vi "Motor controller.vi"() -> ()   [LabVIEW 2015]
uses:
  Power control/Power control.lvclass
  <vilib>/Utility/config.llb/Write Key (Double).vi
  <vilib>/Utility/config.llb/Write Key (String).vi
  <vilib>/Utility/config.llb/Write Key (Boolean).vi
  <vilib>/Utility/config.llb/Write Key (I32).vi
  <vilib>/Utility/config.llb/Read Key (Double).vi
  <vilib>/Utility/config.llb/Read Key (String).vi
  <vilib>/Utility/config.llb/Read Key (Boolean).vi
  <vilib>/Utility/config.llb/Read Key (I32).vi
  Motor controller/Motor/Motor.lvclass
  Motor controller/Signaller/Signaller.lvclass
  Motor controller/Automatic mode/Automatic Mode.lvclass
  Motor controller/Motor/AlphaStep One/AlphaStep One.lvclass
  Motor controller/Motor/Dummy Motor/Dummy Motor.lvclass
  <vilib>/Utility/config.llb/NI_LVConfig.lvlib
  Position-Tracker/x64/Release/PositionTrackerDll.dll
  Motor-Tracker/Release/x64/MotorTrackerDll.dll
panel:
  out "error out":errorcluster
  out "Calculated\nFrequency":dbl
  in  "Show advanced configuration":bool
  in  "Tab Control":enum32{"Advanced configuration"}(tab)
  in  "Reseek after # bad":u32=4
  in  "Samples per step":i32=3 min=0
  in  "\"Good\" rate threshold":dbl=0.8 min=0.0
  out "Countdown overridden":bool
  in  "Algorithm switch time (min)":i64=10 min=0
  out "Automatic mode start":timestamp
  in  "0.01 GHz/step":bool
  in  "0.05 GHz/step":bool
  in  "0.03 GHz/step":bool
  in  "Reset everything":bool
  in  "Make up fit parameters":bool
  in  "Automatic velocity (rev/sec)":dbl=0.1 min=0.0 max=1.0
  in  "Reseek":bool
  in  "Automatic step size (rev)":dbl=0.01 min=0.0 max=1.0
  in  "Reset countdown":bool
  out "Polarization switch countdown":string="0:00"
  in  "Polarization seek":bool
  in  "Home frequency":cluster{"Positive":dbl, "Negative":dbl}={"Positive"=140.18, "Negative"=140.45} {"Negative" format="%.3g"; "Positive" format="%.3g"}
  in  "Negative seek bounds":cluster{"Minimum":dbl, "Maximum":dbl}={"Minimum"=140.35, "Maximum"=140.65} {"Maximum" format="%.3g"; "Minimum" format="%.3g"}
  in  "Positive seek bounds":cluster{"Minimum":dbl, "Maximum":dbl}={"Minimum"=140.1, "Maximum"=140.3} {"Maximum" format="%.3g"; "Minimum" format="%.3g"}
  in  "Seek positive polarization":bool=TRUE
  in  "Launch simulation":bool
  out "Polarization":dbl
  out "Eventnum":i64
  out "Samples taken":i32
  out "Rate":dbl
  in  "Data input file":path
  in  "Automatic mode on/off":bool
  in  "Add power reading":bool
  in  "Width (GHz)":dbl=0.05 format="%.3g"
  in  "New power (mW)":dbl=1.0 format="%.3g"
  out "Microwave power (mW)":dbl format="%.3g"
  in  "Home frequency 2":cluster{"Positive":dbl, "Negative":dbl}={"Positive"=140.18, "Negative"=140.45} {"Negative" format="%.3g"; "Positive" format="%.3g"}
  in  "Debug mode":bool
  in  "Stop communication":bool
  in  "COM Port":refnum<visa-resource-name>
  in  "Step size (GHz)":dbl min=0.0 max=1.0 step=0.001 format="%.3g"
  in  "Goto frequency":bool
  in  "Frequency to seek (GHz)":dbl format="%.3g"
  in  "Stop motor":bool
  in  "Move up":bool
  in  "Move down":bool
  in  "Velocity (rev/sec)":dbl min=0.0 max=1.0 step=0.001
  in  "Step size (rev)":dbl=0.01 min=0.0 max=5.0 step=0.001 format="%.3g"
  in  "Restore configuration from file":bool
  in  "Save configuration to file":bool
  in  "Refine fit parameters":bool
  out "Fit parameters":cluster{"Slope":dbl, "Intercept":dbl}
  in  "Calculate fit parameters":bool
  in  "Read position 2":bool
  in  "Read position 1":bool
  out "Position 2":dbl
  in  "Frequency 2":dbl=140.4 min=0.0 step=0.001 format="%.3g"
  out "Position 1":dbl
  in  "Frequency 1":dbl=140.0 min=0.0 step=0.001 format="%.3g"
  out "Alarm":bool
  out "Alarm code":i32 format="0x%02x"
  out "Frequency (calculated, GHz)":dbl format="%.3g"
  out "Motor position (rev)":dbl format="%.3g"
  out "Motor time (sec)":dbl
  # "Advanced configuration"
  # "Step size presets"
  # "Automatic control"
  # "Power data"
  # "Communication setup"
  # "Please wait after stopping the VI; it can take some time to shut down all the stuff running in the background, so please be patient."
  # "Manual motor control"
  # "Configuration backup/restore"
  # "The settings which are backed up by this method are: step size, frequency to seek, fit slope, fit intercept, automatic step size, automatic velocity, data input file, and all the other controls under \"Automatic control\"."
  # "Frequency calibration"
  # "Motor alarm (error)"
  # "See motor manual, section \"Troubleshooting\" for explanation of alarm codes; fix the problem first and then restart this VI"
  # "Motor information"
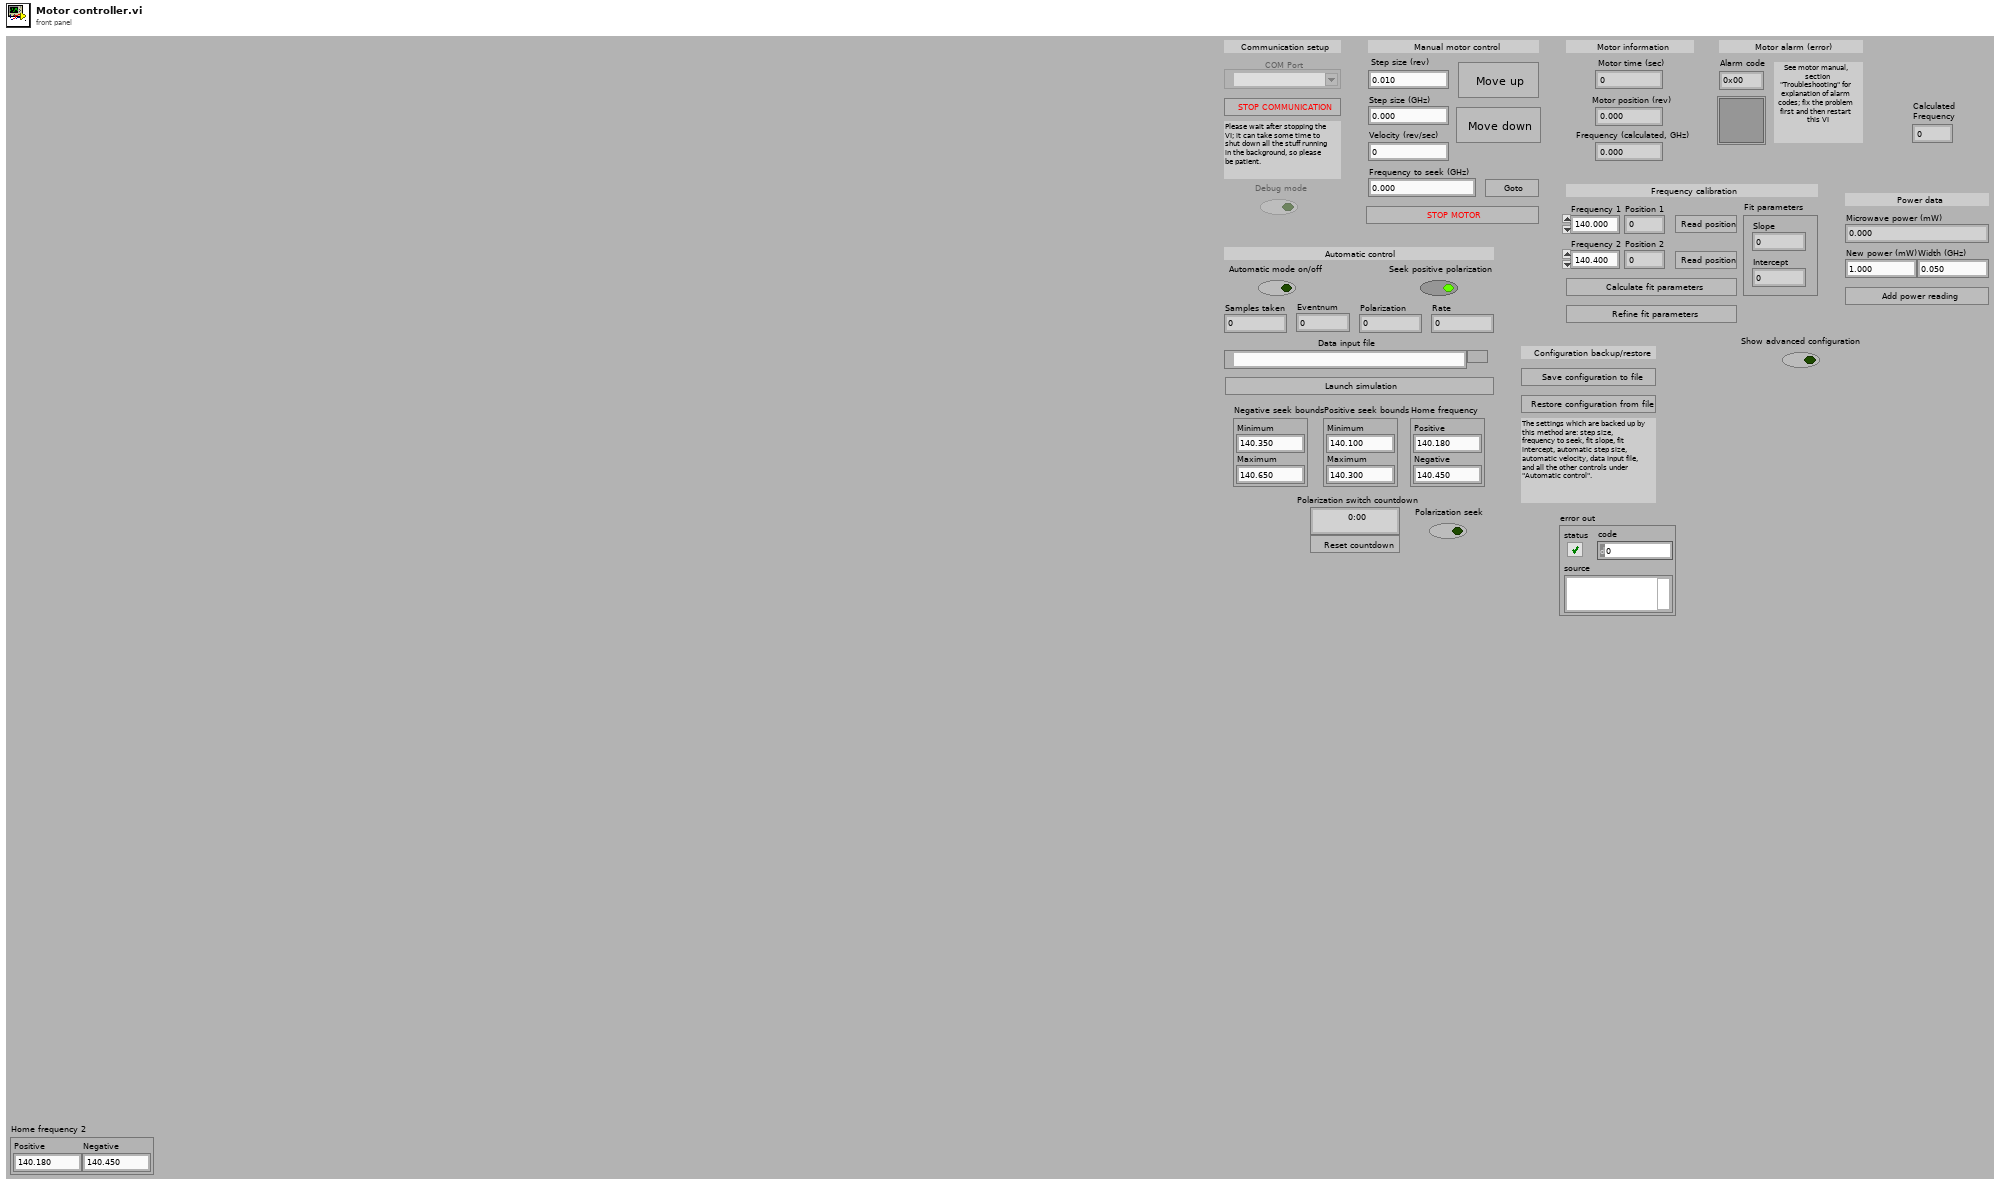
[diagram p1: front panel]
types:
  T1 = enum8{"Enabled", "Disabled", "Disabled and Grayed Out"}
  T2 = typedef "NI_LVConfig.lvlib/Config Data RefNum.ctl" = refnum<k1>
  T3 = typedef "Controller decision.ctl" = enum16{"No motion", "Switch direction", "Keep current direction"}
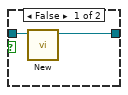
[diagram p2: hidden frame]
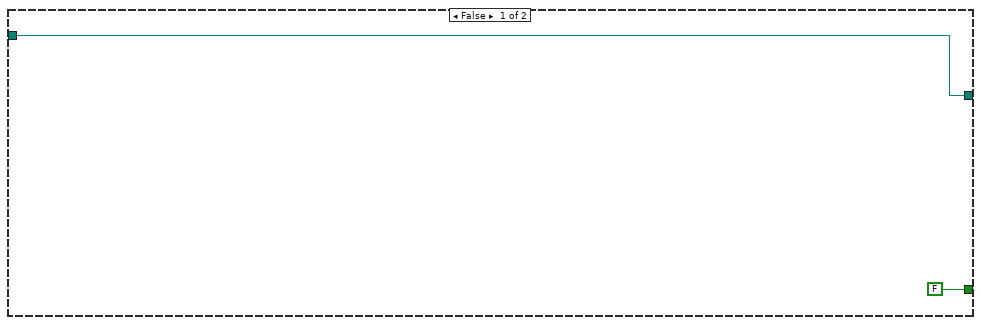
[diagram p5: hidden frame]
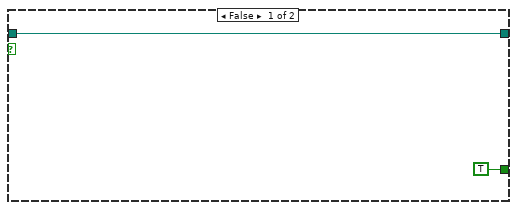
[diagram p6: hidden frame]
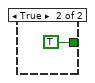
[diagram p7: hidden frame]
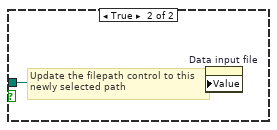
[diagram p8: hidden frame]
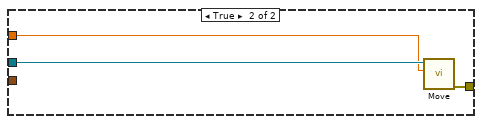
[diagram p12: hidden frame]
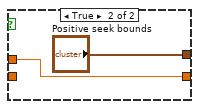
[diagram p13: hidden frame]
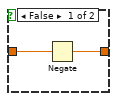
[diagram p14: hidden frame]
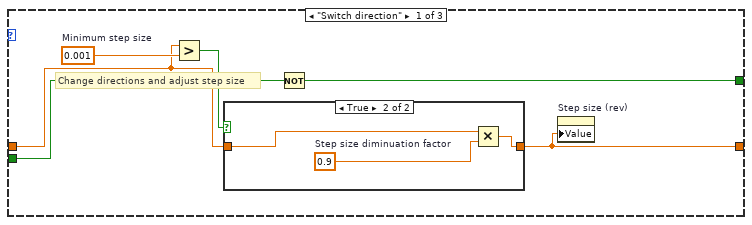
[diagram p15: hidden frame]
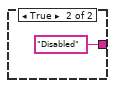
[diagram p18: hidden frame]
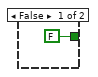
[diagram p20: hidden frame]
diagram:
  w7 = refnum<class "Power control.lvclass"> refnum  # Power control
  w41 = TRUE  # Positive direction?
  (unwired) i64 0
  # "Stop signaller"
  # "Create a new automatic mode object\nto keep track of our data"
  # "Automatic mode loop"
  n1 = Not(x="Debug mode") -> (.not. x?=w34:bool)
  n2 = Equal?(x="COM Port", y=refnum<visa-resource-name> refnum) -> (x = y?=w35:bool)
  n3 = And(x=w35, y=w34) -> (x .and. y?=w36:bool)
  n4 = case shown="True" w36 {
    tunnel: "COM Port" -> [w43 w44]
    tunnel: [w43 w44] -> w32
    frame False {
    }
    frame True {
      # "Make sure that a COM port is\nselected before trying to do\nother stuff; otherwise, bad\nthings will happen"
      n5 = call "Display Message to User5"() -> ("Got it, thanks"=w45:bool)  [unwired: 10 in, 1 out]
      n6 = Stop(stop? (T)=w45) -> ()
    }
  }
  n7 = vi-ref "Grapher.vi"() -> (w12:refnum<vi>)
  n8 = property class="VI Interface Type 3"(reference=w12) -> ("Name"=w13:string)  [unwired: 1 in, 2 out]
  n9 = Open VI Reference(type specifier VI Refnum (for type only)=w12, vi path=w13, options=128) -> (vi reference=w15:refnum<vi>)  [unwired: 3 in, 1 out]
  n10 = vi-ref "Simulation.vi"() -> (w21:refnum<vi>)
  n11 = case shown="True" "Debug mode" {
    tunnel: w32 -> [w47 _]
    tunnel: [w46 w48] -> w2
    frame False {
      n12 = call "New.vi"("VISA resource name"=w47) -> ("AlphaStep One out"=w46:refnum<class "AlphaStep One.lvclass">)  [unwired: 9 in, 1 out]
    }
    frame True {
      n13 = call "New.vi"() -> ("Dummy Motor out"=w48:refnum<class "Dummy Motor.lvclass">)  [unwired: 10 in, 1 out]
    }
  }
  n14 = control-ref of="Frequency (calculated, GHz)"() -> (w17:refnum<vi>)
  n15 = property class="VI Interface Type 2"(reference=w21) -> ("Name"=w22:string)  [unwired: 1 in, 2 out]
  n16 = Obtain Queue "Simulation config action queue"(element data type=cluster{path, bool} {path "", FALSE}) -> (queue out=w8:refnum<queue>)  [unwired: 4 in, 2 out]
  n17 = call-dynamic "Calibrate.vi"("Motor in"=w2) -> ("Motor out"=w1:refnum<class "Motor.lvclass">)  [unwired: 9 in, 1 out]
  n18 = control-ref of="Polarization"() -> (w18:refnum<vi>)
  n19 = control-ref of="Eventnum"() -> (w16:refnum<vi>)
  n20 = control-ref of="Frequency (calculated, GHz)"() -> (w25:refnum<vi>)
  n21 = control-ref of="Rate"() -> (w19:refnum<vi>)
  n22 = New Data Value Reference(data value=w7) -> (data value reference=w6:refnum<data-value>)  [unwired: 1 in, 1 out]
  n23 = Open VI Reference(type specifier VI Refnum (for type only)=w21, vi path=w22, options=128) -> (vi reference=w23:refnum<vi>)  [unwired: 3 in, 1 out]
  n24 = control-ref of="Data input file"() -> (w24:refnum<vi>)
  n25 = call-dynamic "Get velocity.vi"("Motor in"=w1) -> ("error out"=w30:errorcluster, "Velocity (rev/sec)"=w31:dbl, "Motor out"=w29:refnum<class "Motor.lvclass">)  [unwired: 8 in]
  n26 = call "New.vi"("Reseek after # bad polarizations (4)"="Reseek after # bad", "Number of samples (3)"="Samples per step") -> ("Automatic Mode out"=w37:refnum<class "Automatic Mode.lvclass">)  [unwired: 8 in, 1 out]
  n27 = property on="Velocity (rev/sec)" class="DigNum (strict)"("Value"=w31) -> ()  [unwired: 2 in, 2 out]
  n28 = call "New.vi"() -> ("Signaller out"=w10:refnum<class "Signaller.lvclass">)  [unwired: 11 in]
  n29 = call-by-ref "Start Asynchronous Call"(reference=w15, "Eventnum refnum"=w16, "Frequency refnum"=w17, "Stop signaller"=w10, "Polarization refnum"=w18, "Rate refnum"=w19) -> (reference out=w11:refnum<vi>)  [unwired: 12 in, 1 out]
  n30 = call-by-ref "Start Asynchronous Call"(reference=w23, "Stop signaller"=w10, "Simulation config action queue"=w8, "Frequency refnum"=w25, "Data input file refnum"=w24) -> (reference out=w20:refnum<vi>)  [unwired: 2 in, 1 out]
  n31 = Unbundle By Name(w30) -> ("status"=w33:bool)
  n32 = while {
    tunnel: w10 -> [w69]
    tunnel: w6 -> [w65]
    stop <- w68 stop-if-true
    # "Loop for updating user interface objects,\nthat is, things which require no serial\ncommunication"
    n33 = call "Peek or default.vi"("Signaller in"=w69) -> ("Has signal?"=w68:bool)  [unwired: 8 in, 2 out]
    n34 = property on="Automatic mode start" class="AbsTime (strict)"() -> ("Value"=w50:timestamp)  [unwired: 2 in, 2 out]
    n35 = property on="Alarm code" class="DigNum (strict)"() -> ("Value"=w67:i32)  [unwired: 2 in, 2 out]
    n36 = property on="Motor position (rev)" class="DigNum (strict)"() -> ("Value"=w70:dbl)  [unwired: 2 in, 2 out]
    n37 = property on="Fit parameters" class="Clust (strict)"() -> ("Value"=w71:cluster{"Slope":dbl, "Intercept":dbl})  [unwired: 2 in, 2 out]
    n38 = property on="Countdown overridden" class="Bool (strict)"() -> ("Value"=w57:bool)  [unwired: 2 in, 2 out]
    n39 = Not Equal To 0?(x=w67) -> (x != 0?=w66:bool)
    n40 = Equal To 0?(x=w50) -> (x = 0?=w56:bool)
    n41 = case shown="True" w66 {
      tunnel: [FALSE TRUE] -> w72
      frame False {
      }
      frame True {
        # "Turn on alarm light if there is an alarm"
      }
    }
    "Alarm" <- w72
    n42 = call "Motor position to frequency.vi"("Fit parameters"=w71, "Motor position"=w70) -> ("Frequency"=w64:dbl)  [unwired: 9 in]
    "Frequency (calculated, GHz)" <- w64
    n43 = Get Date/Time In Seconds() -> (seconds since 1Jan1904=w63:timestamp)
    n44 = in-place {
      in-place-border: w64 -> [w81]
      n45 = in-place-dvr #1(w65) -> (w80:refnum<class "Power control.lvclass">)  [unwired: 1 out]
      n46 = call "Get reading.vi"("Frequency (GHz)"=w81, "Power control in"=w80) -> ("Power (mW)"=→"Microwave power (mW)":dbl, "Power control out"=w78:refnum<class "Power control.lvclass">)  [unwired: 7 in, 1 out]
      n47 = in-place-dvr #1(w78) -> ()  [unwired: 2 out]
    }
    n48 = Or(x=w57, y=w56) -> (x .or. y?=w55:bool)
    n49 = call "Time difference.vi"("Start time"=w50, "Current time"=w63) -> ("Difference (sec)"=w52:i64)  [unwired: 9 in]
    n50 = Multiply(x="Algorithm switch time (min)", y=i64 60) -> (x*y=w54:i64)
    n51 = Greater Or Equal?(x=w52, y=w54) -> (x >= y?=w61:bool)
    n52 = Not(x=w57) -> (.not. x?=w59:bool)
    n53 = case shown="False" w55 {
      tunnel: [w75 "Disabled"] -> w58
      tunnel: "Algorithm switch time (min)" -> [w74 _]
      tunnel: w52 -> [w73 _]
      frame False {
        n54 = call "Format countdown.vi"("Elapsed (sec)"=w73, "Countdown total (min)"=w74) -> ("Formatted countdown"=w75:string)  [unwired: 9 in]
      }
      frame True {
      }
    }
    "Polarization switch countdown" <- w58
    n55 = Not Equal To 0?(x=w50) -> (x != 0?=w51:bool)
    n56 = Compound Arithmetic op=AND(w61, w59, w51) -> (w60:bool)
    n57 = case shown="True" w60 {
      frame False {
      }
      frame True {
        n58 = property on="Polarization seek" class="Bool (strict)"("Value"=TRUE ("Polarization seek")) -> ()  [unwired: 2 in, 2 out]
      }
    }
    n59 = property on="Tab Control" class="TabCtl (strict)"("Visible"="Show advanced configuration") -> ()  [unwired: 2 in, 2 out]
  }
  n60 = while {
    tunnel: w29 -> [w100]
    tunnel: w10 -> [w103]
    tunnel: [T1."Enabled" ("Disabled")] -> w3
    stop <- w102 stop-if-true
    w95 = T1."Disabled and Grayed Out" ("Disabled")
    # "But be sure to reenable them\non shutdown"
    # "Since changing these values can't do anything\nwhile the controller is running, we disable them"
    # "Loop for updating data continuously\n(i.e. motor position, alarm status, etc.)"
    # "When automatic mode is enabled, we should disable\nmanual mode controls; when automatic mode is\ndisabled, they should be enabled"
    n61 = call "Peek or default.vi"("Signaller in"=w103) -> ("Has signal?"=w102:bool)  [unwired: 8 in, 2 out]
    n62 = case shown="True" "Automatic mode on/off" {
      tunnel: [T1."Enabled" ("Disabled") T1."Disabled and Grayed Out" ("Disabled")] -> w101
      frame False {
      }
      frame True {
      }
    }
    n63 = call-dynamic "Get uptime.vi"("Motor in"=w100) -> ("Uptime (sec)"=→"Motor time (sec)":dbl, "Motor out"=w87:refnum<class "Motor.lvclass">)  [unwired: 8 in, 1 out]
    n64 = call-dynamic "Get position.vi"("Motor in"=w87) -> ("Position (rev)"=→"Motor position (rev)":dbl, "Motor out"=w98:refnum<class "Motor.lvclass">)  [unwired: 8 in, 1 out]
    n65 = call-dynamic "Check error.vi"("Motor in"=w98) -> ("Error code"=→"Alarm code":i32)  [unwired: 8 in, 2 out]
    n66 = call-dynamic "Get position.vi"("Motor in"=w87) -> ("Position (rev)"=w88:dbl)  [unwired: 8 in, 2 out]
    n67 = dll-call lib="C:/Users/ptgroup/Desktop/Slow-Controls/Motor-Tracker/Release/x64/MotorTrackerDll.dll" fn="?MotorTracker@@YANNPEBD@Z"("position"=w88, "file"="C:\\\\Users\\\\ptgroup\\\\Desktop\\\\Slow-Controls\\\\Motor Controller\\\\motormap.csv") -> (error out=→"error out":errorcluster, "return type"=→"Calculated\nFrequency":dbl)  [unwired: 5 in, 1 out]
    n68 = call-dynamic "Get position.vi"("Motor in"=w87) -> ("Position (rev)"=w93:dbl)  [unwired: 8 in, 2 out]
    n69 = property on="Debug mode" class="Bool (strict)"("DisabledEnum"=w95) -> ()  [unwired: 2 in, 2 out]
    n70 = feedback #2() -> (w91:dbl)  [unwired: 1 in]
    n71 = dll-call lib="C:/Users/ptgroup/Desktop/Slow-Controls/Position-Tracker/x64/Release/PositionTrackerDll.dll" fn="?PositionTracker@@YANNNPEBDH@Z"("position"=w93, "buffer"=w91, "file"="C:\\\\Users\\\\ptgroup\\\\Desktop\\\\Slow-Controls\\\\Motor Controller\\\\position.log", "delay"=10) -> ("position"=w92:dbl)  [unwired: 7 in, 2 out]
    n72 = feedback-in #2(w92) -> ()
    n73 = property on="COM Port" class="VISAName"("DisabledEnum"=w95) -> ()  [unwired: 2 in, 2 out]
    n74 = property on="Samples per step" class="DigNum (strict)"("DisabledEnum"=w95) -> ()  [unwired: 2 in, 2 out]
    n75 = property on="Reseek after # bad" class="DigNum (strict)"("DisabledEnum"=w95) -> ()  [unwired: 2 in, 2 out]
    n76 = property on="Stop motor" class="Bool"("DisabledEnum"=w101) -> ()  [unwired: 2 in, 2 out]
    n77 = property on="Move up" class="Bool"("DisabledEnum"=w101) -> ()  [unwired: 2 in, 2 out]
    n78 = property on="Move down" class="Bool"("DisabledEnum"=w101) -> ()  [unwired: 2 in, 2 out]
    n79 = property on="Goto frequency" class="Bool"("DisabledEnum"=w101) -> ()  [unwired: 2 in, 2 out]
    n80 = property on="Frequency to seek (GHz)" class="DigNum (strict)"("DisabledEnum"=w101) -> ()  [unwired: 2 in, 2 out]
    n81 = property on="Step size (GHz)" class="DigNum (strict)"("DisabledEnum"=w101) -> ()  [unwired: 2 in, 2 out]
    n82 = property on="Step size (rev)" class="DigNum (strict)"("DisabledEnum"=w101) -> ()  [unwired: 2 in, 2 out]
    n83 = property on="Velocity (rev/sec)" class="DigNum (strict)"("DisabledEnum"=w101) -> ()  [unwired: 2 in, 2 out]
  }
  n84 = while {
    tunnel: w29 -> [w111]
    tunnel: w10 -> [w112]
    tunnel: [w112] -> w42
    tunnel: [w111] -> w27
    tunnel: w20 -> [w110]
    tunnel: w11 -> [w109]
    tunnel: w8 -> [w108]
    tunnel: w6 -> [w107]
    stop <- w114 stop-if-true
    # "This loop (and all others) will stop executing\nonce the stop notification queue gets a notification\ntelling it to stop (handled by the \"stop on notification\"\nsubVI)"
    # "Event loop; should handle all user-facing events\n(button presses, changing the motor velocity, etc.)"
    n85 = call "Peek or default.vi"("Signaller in"=w112) -> ("Has signal?"=w114:bool)  [unwired: 8 in, 2 out]
    n86 = event shown="[1] \"Move down\": Value Change" {
      selector: _ -> [_ _ _ _ _ _ _ _ _ _ _ _ _ _ _ _ _ _ _ _ _ _ _ _ _ _ _]
      dyn-events: _ -> [_ _ _ _ _ _ _ _ _ _ _ _ _ _ _ _ _ _ _ _ _ _ _ _ _ _ _]
      timeout: 50 -> [_ _ _ _ _ _ _ _ _ _ _ _ _ _ _ _ _ _ _ _ _ _ _ _ _ _ _]
      tunnel: w111 -> [w115 w117 _ _ w132 w134 w154 _ _ _ _ _ _ _ w238 w257 _ _ _ _ _ _ _ _ _ w491 _]
      tunnel: w112 -> [_ _ _ _ _ _ _ _ _ _ _ _ _ _ _ _ _ _ _ _ _ _ _ _ w486 w494 _]
      tunnel: w110 -> [_ _ _ _ _ _ _ _ _ _ _ _ w226 _ _ _ _ _ _ _ _ _ _ _ _ _ _]
      tunnel: w109 -> [_ _ _ _ _ _ _ _ _ _ _ _ _ _ w237 _ _ _ _ _ _ _ _ _ _ _ _]
      tunnel: w108 -> [_ _ _ _ _ _ _ _ _ _ _ _ _ _ _ _ _ _ _ _ _ _ w298 w376 _ _ _]
      tunnel: w107 -> [_ _ _ _ _ _ _ _ _ _ _ w216 _ _ _ _ _ _ _ _ _ _ w297 w375 _ _ _]
      event "Move up": Value Change {
        n87 = event-data() -> ()  [unwired: 1 in, 5 out]
        n88 = property on="Step size (rev)" class="DigNum (strict)"() -> ("Value"=w116:dbl)  [unwired: 2 in, 2 out]
        n89 = call-dynamic "Move.vi"("Amount (rev)"=w116, "Motor in"=w115) -> ()  [unwired: 8 in, 2 out]
      }
      event "Move down": Value Change {
        n90 = event-data() -> ()  [unwired: 1 in, 5 out]
        n91 = property on="Step size (rev)" class="DigNum (strict)"() -> ("Value"=w119:dbl)  [unwired: 2 in, 2 out]
        n92 = Negate(x=w119) -> (-x=w118:dbl)
        n93 = call-dynamic "Move.vi"("Amount (rev)"=w118, "Motor in"=w117) -> ()  [unwired: 8 in, 2 out]
      }
      event "Step size (rev)": Value Change {
        n94 = event-data() -> ()  [unwired: 1 in, 6 out]
        n95 = property on="Step size (rev)" class="DigNum (strict)"() -> ("Value"=w123:dbl)  [unwired: 2 in, 2 out]
        n96 = property on="Slope" class="DigNum (strict)"() -> ("Value"=w122:dbl)  [unwired: 2 in, 2 out]
        n97 = Multiply(x=w123, y=w122) -> (x*y=w121:dbl)
        n98 = Absolute Value(x=w121) -> (abs(x)=w120:dbl)
        n99 = property on="Step size (GHz)" class="DigNum (strict)"("Value"=w120) -> ()  [unwired: 2 in, 2 out]
      }
      event "Step size (GHz)": Value Change {
        n100 = event-data() -> ()  [unwired: 1 in, 6 out]
        n101 = property on="Slope" class="DigNum (strict)"() -> ("Value"=w124:dbl)  [unwired: 2 in, 2 out]
        n102 = Not Equal To 0?(x=w124) -> (x != 0?=w126:bool)
        n103 = case shown="True" w126 {
          tunnel: "Step size (GHz)" -> [_ w130]
          tunnel: w124 -> [_ w129]
          frame False {
            n104 = call "Display Message to User15"() -> ()  [unwired: 10 in, 2 out]
          }
          frame True {
            n105 = Divide(x=w130, y=w129) -> (x/y=w128:dbl)
            n106 = Absolute Value(x=w128) -> (abs(x)=w127:dbl)
            n107 = property on="Step size (rev)" class="DigNum (strict)"("Value"=w127) -> ()  [unwired: 2 in, 2 out]
          }
        }
      }
      event "Velocity (rev/sec)": Value Change {
        n108 = event-data() -> ()  [unwired: 1 in, 5 out]
        n109 = call-dynamic "Set velocity.vi"("Velocity (rev/sec)"="Velocity (rev/sec)", "Motor in"=w132) -> ()  [unwired: 8 in, 2 out]
      }
      event "Goto frequency": Value Change {
        n110 = event-data() -> ()  [unwired: 1 in, 5 out]
        n111 = property on="Fit parameters" class="Clust (strict)"() -> ("Value"=w133:cluster{"Slope":dbl, "Intercept":dbl})  [unwired: 2 in, 2 out]
        n112 = Unbundle By Name(w133) -> ("Slope"=w135:dbl)
        n113 = Equal To 0?(x=w135) -> (x = 0?=w136:bool)
        n114 = case shown="False" w136 {
          tunnel: w134 -> [w145 _]
          tunnel: w133 -> [w138 _]
          frame False {
            # "Calculate corresponding motor position and go there"
            n115 = property on="Motor position (rev)" class="DigNum (strict)"() -> ("Value"=w146:dbl)  [unwired: 2 in, 2 out]
            n116 = call "Frequency to motor position.vi"("Fit parameters"=w138, "Frequency"="Frequency to seek (GHz)") -> ("Motor position"=w137:dbl)  [unwired: 9 in]
            n117 = Subtract(x=w137, y=w146) -> (x-y=w143:dbl)
            n118 = Absolute Value(x=w143) -> (abs(x)=w142:dbl)
            n119 = Less?(x=w142, y=1.0) -> (x < y?=w139:bool)
            n120 = case shown="False" w139 {
              selector: w139 -> [_ w151]
              tunnel: [w147 w151] -> w140
              frame False {
                n121 = Two Button Dialog(message="The frequency you are attempting to go to is very far from the current position; you may run into problems. Are you sure you want to continue?", 1:"No" ("F button name (\"Cancel\")"), 2:"Yes" ("T button name (\"OK\")")) -> (T button?=w147:bool)
              }
              frame True {
              }
            }
            n122 = case shown="True" w140 {
              tunnel: w145 -> [_ w152]
              tunnel: w137 -> [_ w153]
              frame False {
              }
              frame True {
                n123 = call-dynamic "Move to position.vi"("Position"=w153, "Motor in"=w152) -> ()  [unwired: 8 in, 2 out]
              }
            }
          }
          frame True {
            n124 = call "Display Message to User"() -> ()  [unwired: 10 in, 2 out]
          }
        }
      }
      event "Stop motor": Value Change {
        n125 = event-data() -> ()  [unwired: 1 in, 5 out]
        n126 = call-dynamic "Stop.vi"("Motor in"=w154) -> ()  [unwired: 9 in, 2 out]
      }
      event "Read position 1": Value Change {
        n127 = event-data() -> ()  [unwired: 1 in, 5 out]
        n128 = property on="Motor position (rev)" class="DigNum (strict)"() -> ("Value"=→"Position 1":dbl)  [unwired: 2 in, 2 out]
      }
      event "Read position 2": Value Change {
        n129 = event-data() -> ()  [unwired: 1 in, 5 out]
        n130 = property on="Motor position (rev)" class="DigNum (strict)"() -> ("Value"=→"Position 2":dbl)  [unwired: 2 in, 2 out]
      }
      event "Calculate fit parameters": Value Change {
        n131 = event-data() -> ()  [unwired: 1 in, 5 out]
        n132 = property on="Position 1" class="DigNum (strict)"() -> ("Value"=w161:dbl)  [unwired: 2 in, 2 out]
        n133 = property on="Position 2" class="DigNum (strict)"() -> ("Value"=w160:dbl)  [unwired: 2 in, 2 out]
        n134 = property on="Calculate fit parameters" class="Bool (strict)"("Value"=FALSE ("Calculate fit parameters")) -> ()  [unwired: 2 in, 2 out]
        n135 = Equal?(x=w161, y=w160) -> (x = y?=w163:bool)
        n136 = Equal?(x="Frequency 1", y="Frequency 2") -> (x = y?=w162:bool)
        n137 = Or(x=w163, y=w162) -> (x .or. y?=w157:bool)
        n138 = case shown="False" w157 {
          tunnel: w161 -> [w172 _]
          tunnel: w160 -> [w171 _]
          tunnel: "Frequency 1" -> [w170 _]
          tunnel: "Frequency 2" -> [w169 _]
          frame False {
            # "Calculate slope and intercept"
            # "The automatic step size should be around 0.02GHz\ninitially, to get a good seek"
            n139 = call "Calculate fit parameters.vi"("Frequency 2"=w169, "Frequency 1"=w170, "Position 2"=w171, "Position 1"=w172) -> ("Intercept"=w173:dbl, "Slope"=w167:dbl)
            n140 = property on="Fit parameters" class="Clust (strict)"() -> ("Value"=w175:cluster{"Slope":dbl, "Intercept":dbl})  [unwired: 2 in, 2 out]
            n141 = Divide(x=0.02, y=w167) -> (x/y=w166:dbl)
            n142 = Bundle By Name(cluster=w175, "Slope"=w167, "Intercept"=w173) -> (→"Fit parameters":cluster{"Slope":dbl, "Intercept":dbl})
            n143 = Absolute Value(x=w166) -> (abs(x)=w165:dbl)
            n144 = property on="Automatic step size (rev)" class="DigNum (strict)"("Value"=w165) -> ()  [unwired: 2 in, 2 out]
          }
          frame True {
            # "Warn the user about trying to calculate/refine\nfit parameters with invalid inputs (fit function\nMUST be bijective; i.e. slope must not be 0\nor infinity)"
            n145 = call "Display Message to User6"() -> ()  [unwired: 10 in, 2 out]
          }
        }
      }
      event "Refine fit parameters": Value Change {
        n146 = event-data() -> ()  [unwired: 1 in, 6 out]
        n147 = property on="Fit parameters" class="Clust (strict)"() -> ("Value"=w181:cluster{"Slope":dbl, "Intercept":dbl})  [unwired: 2 in, 2 out]
        n148 = Unbundle By Name(w181) -> ("Slope"=w177:dbl, "Intercept"=w176:dbl)
        n149 = Equal To 0?(x=w177) -> (x = 0?=w179:bool)
        n150 = Equal To 0?(x=w176) -> (x = 0?=w178:bool)
        n151 = property on="Frequency 1" class="DigNum (strict)"() -> ("Value"=w185:dbl)  [unwired: 2 in, 2 out]
        n152 = property on="Frequency 2" class="DigNum (strict)"() -> ("Value"=w184:dbl)  [unwired: 2 in, 2 out]
        n153 = And(x=w178, y=w179) -> (x .and. y?=w180:bool)
        n154 = property on="Position 2" class="DigNum (strict)"() -> ("Value"=w182:dbl)  [unwired: 2 in, 2 out]
        n155 = property on="Position 1" class="DigNum (strict)"() -> ("Value"=w183:dbl)  [unwired: 2 in, 2 out]
        n156 = case shown="False" w180 {
          tunnel: w185 -> [w187 _]
          tunnel: w184 -> [w186 _]
          tunnel: w183 -> [w192 _]
          tunnel: w182 -> [w191 _]
          tunnel: w177 -> [w195 _]
          tunnel: w176 -> [w194 _]
          tunnel: w181 -> [w193 _]
          frame False {
            n157 = Equal?(x=w192, y=w191) -> (x = y?=w190:bool)
            n158 = Equal?(x=w187, y=w186) -> (x = y?=w189:bool)
            n159 = Or(x=w190, y=w189) -> (x .or. y?=w188:bool)
            n160 = case shown="False" w188 {
              tunnel: w187 -> [w214 _]
              tunnel: w186 -> [w213 _]
              tunnel: w192 -> [w212 _]
              tunnel: w191 -> [w211 _]
              tunnel: w195 -> [w209 _]
              tunnel: w194 -> [w207 _]
              tunnel: w193 -> [w201 _]
              frame False {
                # "Update automatic step size as well,\nas with the \"calculate fit parameters\"\naction"
                # "Average new slope and intercept with\nold ones, to get better approximation"
                n161 = call "Calculate fit parameters.vi"("Frequency 2"=w213, "Frequency 1"=w214, "Position 2"=w211, "Position 1"=w212) -> ("Intercept"=w208:dbl, "Slope"=w210:dbl)
                n162 = Add(x=w210, y=w209) -> (x+y=w206:dbl)
                n163 = Add(x=w208, y=w207) -> (x+y=w205:dbl)
                n164 = Divide(x=w206, y=2.0) -> (x/y=w198:dbl)
                n165 = Divide(x=w205, y=2.0) -> (x/y=w200:dbl)
                n166 = Bundle By Name(cluster=w201, "Slope"=w198, "Intercept"=w200) -> (w202:cluster{"Slope":dbl, "Intercept":dbl})
                n167 = Divide(x=0.02, y=w198) -> (x/y=w197:dbl)
                n168 = Absolute Value(x=w197) -> (abs(x)=w196:dbl)
                n169 = property on="Fit parameters" class="Clust (strict)"("Value"=w202) -> ()  [unwired: 2 in, 2 out]
                n170 = property on="Automatic step size (rev)" class="DigNum (strict)"("Value"=w196) -> ()  [unwired: 2 in, 2 out]
              }
              frame True {
                # "Warn the user about trying to calculate/refine\nfit parameters with invalid inputs (fit function\nMUST be bijective; i.e. slope must not be 0\nor infinity)"
                n171 = call "Display Message to User7"() -> ()  [unwired: 10 in, 2 out]
              }
            }
          }
          frame True {
            # "Warn the user about refining fit parameters\nwithout calculating initial parameters first"
            n172 = call "Display Message to User4"() -> ()  [unwired: 10 in, 2 out]
          }
        }
      }
      event "Add power reading": Value Change {
        n173 = event-data() -> ()  [unwired: 1 in, 6 out]
        n174 = property on="Frequency (calculated, GHz)" class="DigNum (strict)"() -> ("Value"=w215:dbl)  [unwired: 2 in, 2 out]
        n175 = Not Equal To 0?(x=w215) -> (x != 0?=w217:bool)
        n176 = case shown="True" w217 {
          tunnel: w216 -> [_ w219]
          tunnel: w215 -> [_ w218]
          frame False {
            n177 = call "Display Message to User18"() -> ()  [unwired: 10 in, 2 out]
          }
          frame True {
            n178 = in-place {
              in-place-border: w218 -> [w224]
              n179 = in-place-dvr #3(w219) -> (w225:refnum<class "Power control.lvclass">, w221:errorcluster)
              n180 = call "Add reading.vi"("Power (mW)"="New power (mW)", "error in (no error)"=w221, "Width (GHz)"="Width (GHz)", "Frequency (GHz)"=w224, "Power control in"=w225) -> ("Power control out"=w220:refnum<class "Power control.lvclass">)  [unwired: 5 in, 1 out]
              n181 = in-place-dvr #3(w220) -> ()  [unwired: 2 out]
            }
          }
        }
      }
      event "Launch simulation": Value Change {
        # "Tell the simulation notifier to launch the simulation"
        n182 = event-data() -> ()  [unwired: 1 in, 5 out]
        n183 = property on="Fit parameters" class="Clust (strict)"() -> ("Value"=w229:cluster{"Slope":dbl, "Intercept":dbl})  [unwired: 2 in, 2 out]
        n184 = Unbundle By Name(w229) -> ("Slope"=w228:dbl)
        n185 = Equal To 0?(x=w228) -> (x = 0?=w227:bool)
        n186 = case shown="False" w227 {
          tunnel: w226 -> [w230 _]
          frame False {
            n187 = invoke class="VI Interface Type 1" method="FP.Open"(reference=w230) -> ()  [unwired: 4 in, 5 out]
          }
          frame True {
            n188 = call "Display Message to User3"() -> ()  [unwired: 10 in, 2 out]
          }
        }
      }
      event "Reseek": Value Change {
        n189 = event-data() -> ()  [unwired: 1 in, 5 out]
        n190 = property on="Automatic mode on/off" class="Bool (strict)"() -> ("Value"=w234:bool)  [unwired: 2 in, 2 out]
        n191 = And(x=w234, y="Reseek") -> (x .and. y?=w232:bool)
        n192 = property on="Reseek" class="Bool (strict)"("Value"=FALSE ("Reseek")) -> ()  [unwired: 2 in, 2 out]
        n193 = case shown="True" w232 {
          frame False {
          }
          frame True {
            # "Switch back to rate seek and reset countdown."
            # "Change step size back to the default (initial) automatic step size"
            n194 = property on="Automatic step size (rev)" class="DigNum (strict)"() -> ("Value"=w236:dbl)  [unwired: 2 in, 2 out]
            n195 = property on="Reset countdown" class="Bool (strict)"("Val(Sgnl)"=TRUE ("Value (Signaling)")) -> ()  [unwired: 2 in, 2 out]
            n196 = property on="Step size (rev)" class="DigNum (strict)"("Val(Sgnl)"=w236) -> ()  [unwired: 2 in, 2 out]
          }
        }
      }
      event "Automatic mode on/off": Value Change {
        # "When automatic mode is enabled,\nchoose the initial step size and start\ngrapher subvi"
        n197 = event-data() -> ()  [unwired: 1 in, 5 out]
        n198 = property on="Automatic mode on/off" class="Bool (strict)"() -> ("Value"=w239:bool)  [unwired: 2 in, 2 out]
        n199 = case shown="True" w239 {
          tunnel: w238 -> [_ w247]
          tunnel: w237 -> [_ w243]
          frame False {
          }
          frame True {
            # "We only want to set the start time once, so that automatic mode can be temporarily disabled and then re-enabled without changing the algorithm again."
            # "Move to home position"
            n200 = invoke class="VI Interface Type 0" method="FP.Open"(reference=w243) -> ()  [unwired: 4 in, 5 out]
            n201 = property on="Automatic mode start" class="AbsTime (strict)"() -> ("Value"=w242:timestamp)  [unwired: 2 in, 2 out]
            n202 = property on="Seek positive polarization" class="Bool (strict)"() -> ("Value"=w249:bool)  [unwired: 2 in, 2 out]
            n203 = Equal?(x=w242, y=timestamp(0 s since 1904-01-01)) -> (x = y?=w240:bool)
            n204 = property on="Step size (rev)" class="DigNum (strict)"("Val(Sgnl)"="Automatic step size (rev)") -> ()  [unwired: 2 in, 2 out]
            n205 = case shown="True" w240 {
              frame False {
              }
              frame True {
                n206 = Get Date/Time In Seconds() -> (seconds since 1Jan1904=→"Automatic mode start":timestamp)
              }
            }
            n207 = case shown="False" w249 {
              tunnel: "Home frequency" -> [w254 w256]
              tunnel: [w253 w255] -> w246
              frame False {
                n208 = Unbundle By Name(w254) -> ("Negative"=w253:dbl)
              }
              frame True {
                n209 = Unbundle By Name(w256) -> ("Positive"=w255:dbl)
              }
            }
            n210 = property on="Velocity (rev/sec)" class="DigNum (strict)"("Val(Sgnl)"="Automatic velocity (rev/sec)") -> ()  [unwired: 2 in, 2 out]
            n211 = property on="Fit parameters" class="Clust (strict)"() -> ("Value"=w244:cluster{"Slope":dbl, "Intercept":dbl})  [unwired: 2 in, 2 out]
            n212 = call "Frequency to motor position.vi"("Fit parameters"=w244, "Frequency"=w246) -> ("Motor position"=w245:dbl)  [unwired: 9 in]
            n213 = call-dynamic "Move to position.vi"("Position"=w245, "Motor in"=w247) -> ()  [unwired: 8 in, 2 out]
          }
        }
      }
      event "Seek positive polarization": Value Change {
        # "Move to home position"
        n214 = event-data() -> ()  [unwired: 1 in, 6 out]
        n215 = property on="Seek positive polarization" class="Bool (strict)"() -> ("Value"=w259:bool)  [unwired: 2 in, 2 out]
        n216 = case shown="False" w259 {
          tunnel: "Home frequency 2" -> [w264 w266]
          tunnel: [w263 w265] -> w261
          frame False {
            n217 = Unbundle By Name(w264) -> ("Negative"=w263:dbl)
          }
          frame True {
            n218 = Unbundle By Name(w266) -> ("Positive"=w265:dbl)
          }
        }
        n219 = property on="Fit parameters" class="Clust (strict)"() -> ("Value"=w258:cluster{"Slope":dbl, "Intercept":dbl})  [unwired: 2 in, 2 out]
        n220 = call "Frequency to motor position.vi"("Fit parameters"=w258, "Frequency"=w261) -> ("Motor position"=w260:dbl)  [unwired: 9 in]
        n221 = call-dynamic "Move to position.vi"("Position"=w260, "Motor in"=w257) -> ()  [unwired: 8 in, 2 out]
      }
      event "Polarization seek": Value Change {
        n222 = event-data() -> ()  [unwired: 1 in, 6 out]
        "Countdown overridden" <- TRUE ("Countdown overridden")
      }
      event "Reset countdown": Value Change {
        n223 = event-data() -> ()  [unwired: 1 in, 6 out]
        n224 = case shown="True" "Reset countdown" {
          frame False {
          }
          frame True {
            n225 = Get Date/Time In Seconds() -> (seconds since 1Jan1904=w272:timestamp)
            n226 = property on="Automatic mode start" class="AbsTime (strict)"("Value"=w272) -> ()  [unwired: 2 in, 2 out]
            n227 = property on="Countdown overridden" class="Bool (strict)"("Value"=FALSE ("Countdown overridden")) -> ()  [unwired: 2 in, 2 out]
            n228 = property on="Polarization seek" class="Bool (strict)"("Value"=FALSE ("Polarization seek")) -> ()  [unwired: 2 in, 2 out]
            n229 = property on="Reset countdown" class="Bool (strict)"("Value"=FALSE ("Reset countdown")) -> ()  [unwired: 2 in, 2 out]
          }
        }
      }
      event "0.05 GHz/step": Value Change {
        n230 = event-data() -> ()  [unwired: 1 in, 6 out]
        n231 = property on="Slope" class="DigNum (strict)"() -> ("Value"=w273:dbl)  [unwired: 2 in, 2 out]
        n232 = Not Equal To 0?(x=w273) -> (x != 0?=w274:bool)
        n233 = case shown="True" w274 {
          tunnel: w273 -> [_ w277]
          frame False {
            n234 = call "Display Message to User12"() -> ()  [unwired: 10 in, 2 out]
          }
          frame True {
            n235 = Divide(x=0.05, y=w277) -> (x/y=w276:dbl)
            n236 = Absolute Value(x=w276) -> (abs(x)=w275:dbl)
            n237 = property on="Automatic step size (rev)" class="DigNum (strict)"("Value"=w275) -> ()  [unwired: 2 in, 2 out]
          }
        }
      }
      event "0.03 GHz/step": Value Change {
        n238 = event-data() -> ()  [unwired: 1 in, 6 out]
        n239 = property on="Slope" class="DigNum (strict)"() -> ("Value"=w279:dbl)  [unwired: 2 in, 2 out]
        n240 = Not Equal To 0?(x=w279) -> (x != 0?=w280:bool)
        n241 = case shown="True" w280 {
          tunnel: w279 -> [_ w283]
          frame False {
            n242 = call "Display Message to User13"() -> ()  [unwired: 10 in, 2 out]
          }
          frame True {
            n243 = Divide(x=0.03, y=w283) -> (x/y=w282:dbl)
            n244 = Absolute Value(x=w282) -> (abs(x)=w281:dbl)
            n245 = property on="Automatic step size (rev)" class="DigNum (strict)"("Value"=w281) -> ()  [unwired: 2 in, 2 out]
          }
        }
      }
      event "0.01 GHz/step": Value Change {
        n246 = event-data() -> ()  [unwired: 1 in, 6 out]
        n247 = property on="Slope" class="DigNum (strict)"() -> ("Value"=w285:dbl)  [unwired: 2 in, 2 out]
        n248 = Not Equal To 0?(x=w285) -> (x != 0?=w286:bool)
        n249 = case shown="True" w286 {
          tunnel: w285 -> [_ w289]
          frame False {
            n250 = call "Display Message to User14"() -> ()  [unwired: 10 in, 2 out]
          }
          frame True {
            n251 = Divide(x=0.01, y=w289) -> (x/y=w288:dbl)
            n252 = Absolute Value(x=w288) -> (abs(x)=w287:dbl)
            n253 = property on="Automatic step size (rev)" class="DigNum (strict)"("Value"=w287) -> ()  [unwired: 2 in, 2 out]
          }
        }
      }
      event "Make up fit parameters": Value Change {
        # "Make up some fit parameters (no physical meaning)\nfor quick testing of automatic mode"
        n254 = event-data() -> ()  [unwired: 1 in, 5 out]
        n255 = flat-sequence {
          frame #0 {
            n256 = property on="Frequency 2" class="DigNum (strict)"("Value"=140.15 ("Frequency 2")) -> ()  [unwired: 2 in, 2 out]
            n257 = property on="Frequency 1" class="DigNum (strict)"("Value"=140.1 ("Frequency 1")) -> ()  [unwired: 2 in, 2 out]
            n258 = property on="Motor position (rev)" class="DigNum (strict)"() -> ("Value"=w295:dbl)  [unwired: 2 in, 2 out]
            n259 = property on="Position 2" class="DigNum (strict)"("Value"=w295) -> ()  [unwired: 2 in, 2 out]
            n260 = property on="Step size (rev)" class="DigNum (strict)"() -> ("Value"=w293:dbl)  [unwired: 2 in, 2 out]
            n261 = Subtract(x=w295, y=w293) -> (x-y=w294:dbl)
            n262 = property on="Position 1" class="DigNum (strict)"("Value"=w294) -> ()  [unwired: 2 in, 2 out]
          }
          frame #1 {
            n263 = property on="Calculate fit parameters" class="Bool (strict)"("Val(Sgnl)"=TRUE ("Value (Signaling)")) -> ()  [unwired: 2 in, 2 out]
          }
        }
      }
      event "Save configuration to file": Value Change {
        # "Ignore error"
        n264 = event-data() -> ()  [unwired: 1 in, 6 out]
        n265 = call "File Dialog"("prompt"="Select file to store configuration", "default name"="controller_settings.ini") -> ("selected path"=w304:path, "exists"=w305:bool, "cancelled"=w302:bool, "error out"=w300:errorcluster)  [unwired: 10 in]
        n266 = Unbundle By Name(w300) -> ()  [unwired: 1 out]
        n267 = Not A Number/Path/Refnum?(number/path/refnum=w304) -> (NaN/Path/Refnum?=w303:bool)
        n268 = Or(x=w303, y=w302) -> (x .or. y?=w301:bool)
        n269 = case shown="False" w301 {
          tunnel: w305 -> [w311 _]
          tunnel: w304 -> [w309 _]
          tunnel: w298 -> [w308 _]
          tunnel: w297 -> [w307 _]
          frame False {
            n270 = case shown="True" w311 {
              tunnel: [TRUE ("Yes") w374] -> w310
              frame False {
              }
              frame True {
                n271 = call "Display Message to User9"() -> ("Yes"=w374:bool)  [unwired: 10 in, 1 out]
              }
            }
            n272 = case shown="True" w310 {
              tunnel: w309 -> [_ w369]
              tunnel: w308 -> [_ w325]
              tunnel: w307 -> [_ w319]
              frame False {
              }
              frame True {
                w362 = i16 3 ("precision (6)")
                w312 = "Controller" ("section")
                # "To save the configuration, we use what LabVIEW calls\na \"configuration file\", which is really just an INI file with\na fancy name. As you can see, the interface for working\nwith these in LabVIEW is quite tedious (like everything in\nLabVIEW), but it works."
                # "Save any important configuration"
                n273 = in-place {
                  in-place-border: [w370] -> w318
                  n274 = in-place-dvr #4(w319) -> (w372:refnum<class "Power control.lvclass">)  [unwired: 1 out]
                  n275 = call "To string.vi"("Power control in"=w372) -> ("String"=w370:string, "Power control out"=w371:refnum<class "Power control.lvclass">)  [unwired: 8 in, 1 out]
                  n276 = in-place-dvr #4(w371) -> ()  [unwired: 2 out]
                }
                n277 = property on="Step size (rev)" class="DigNum (strict)"() -> ("Value"=w366:dbl)  [unwired: 2 in, 2 out]
                n278 = call <vilib>:"Open Config Data.vi"("configuration file path"=w369) -> ("refnum"=w368:T2)  [unwired: 8 in, 2 out]
                n279 = property on="Frequency to seek (GHz)" class="DigNum (strict)"() -> ("Value"=w363:dbl)  [unwired: 2 in, 2 out]
                n280 = call-poly <vilib>:"Write Key.vi"("precision (6)"=w362, "section"=w312, "value"=w366, "key"="Step size", "refnum"=w368) -> ("refnum out"=w365:T2)  [unwired: 4 in, 2 out]
                n281 = call-poly <vilib>:"Write Key.vi"("precision (6)"=w362, "section"=w312, "value"=w363, "key"="Frequency to seek", "refnum"=w365) -> ("refnum out"=w361:T2)  [unwired: 4 in, 2 out]
                n282 = property on="Slope" class="DigNum (strict)"() -> ("Value"=w359:dbl)  [unwired: 2 in, 2 out]
                n283 = call-poly <vilib>:"Write Key.vi"("section"=w312, "value"=w359, "key"="Slope", "refnum"=w361) -> ("refnum out"=w358:T2)  [unwired: 5 in, 2 out]
                n284 = property on="Intercept" class="DigNum (strict)"() -> ("Value"=w356:dbl)  [unwired: 2 in, 2 out]
                n285 = property on="Automatic step size (rev)" class="DigNum (strict)"() -> ("Value"=w353:dbl)  [unwired: 2 in, 2 out]
                n286 = property on="Automatic velocity (rev/sec)" class="DigNum (strict)"() -> ("Value"=w350:dbl)  [unwired: 2 in, 2 out]
                n287 = call-poly <vilib>:"Write Key.vi"("section"=w312, "value"=w356, "key"="Intercept", "refnum"=w358) -> ("refnum out"=w355:T2)  [unwired: 5 in, 2 out]
                n288 = call-poly <vilib>:"Write Key.vi"("section"=w312, "value"=w353, "key"="Automatic step size", "refnum"=w355) -> ("refnum out"=w352:T2)  [unwired: 5 in, 2 out]
                n289 = property on="Data input file" class="Path"() -> ("Text.Text"=w347:string)  [unwired: 2 in, 2 out]
                n290 = call-poly <vilib>:"Write Key.vi"("section"=w312, "value"=w350, "key"="Automatic velocity", "refnum"=w352) -> ("refnum out"=w349:T2)  [unwired: 5 in, 2 out]
                n291 = property on="Seek positive polarization" class="Bool (strict)"() -> ("Value"=w344:bool)  [unwired: 2 in, 2 out]
                n292 = call-poly <vilib>:"Write Key.vi"("section"=w312, "value"=w347, "key"="Data input file", "refnum"=w349) -> ("refnum out"=w346:T2)  [unwired: 5 in, 2 out]
                n293 = property on="Positive" class="DigNum (strict)"() -> ("Value"=w327:dbl)  [unwired: 2 in, 2 out]
                n294 = call-poly <vilib>:"Write Key.vi"("section"=w312, "value"=w344, "key"="Seek positive", "refnum"=w346) -> ("refnum out"=w343:T2)  [unwired: 5 in, 2 out]
                n295 = property on="Minimum" class="DigNum (strict)"() -> ("Value"=w331:dbl)  [unwired: 2 in, 2 out]
                n296 = property on="Maximum" class="DigNum (strict)"() -> ("Value"=w328:dbl)  [unwired: 2 in, 2 out]
                n297 = call-poly <vilib>:"Write Key.vi"("section"=w312, "value"=w331, "key"="Negative minimum frequency", "refnum"=w343) -> ("refnum out"=w342:T2)  [unwired: 5 in, 2 out]
                n298 = property on="Maximum" class="DigNum (strict)"() -> ("Value"=w330:dbl)  [unwired: 2 in, 2 out]
                n299 = call-poly <vilib>:"Write Key.vi"("section"=w312, "value"=w330, "key"="Negative maximum frequency", "refnum"=w342) -> ("refnum out"=w341:T2)  [unwired: 5 in, 2 out]
                n300 = property on="Minimum" class="DigNum (strict)"() -> ("Value"=w329:dbl)  [unwired: 2 in, 2 out]
                n301 = call-poly <vilib>:"Write Key.vi"("section"=w312, "value"=w329, "key"="Positive minimum frequency", "refnum"=w341) -> ("refnum out"=w340:T2)  [unwired: 5 in, 2 out]
                n302 = call-poly <vilib>:"Write Key.vi"("section"=w312, "value"=w328, "key"="Positive maximum frequency", "refnum"=w340) -> ("refnum out"=w339:T2)  [unwired: 5 in, 2 out]
                n303 = call-poly <vilib>:"Write Key.vi"("section"=w312, "value"=w327, "key"="Positive home", "refnum"=w339) -> ("refnum out"=w338:T2)  [unwired: 5 in, 2 out]
                n304 = property on="Algorithm switch time (min)" class="DigNum (strict)"() -> ("Value"=w314:i64)  [unwired: 2 in, 2 out]
                n305 = property on="Negative" class="DigNum (strict)"() -> ("Value"=w326:dbl)  [unwired: 2 in, 2 out]
                n306 = call-poly <vilib>:"Write Key.vi"("section"=w312, "value"=w326, "key"="Negative home", "refnum"=w338) -> ("refnum out"=w321:T2)  [unwired: 5 in, 2 out]
                n307 = call-poly <vilib>:"Write Key.vi"("section"=w312, "value"=w318, "key"="Power data", "refnum"=w321) -> ("refnum out"=w317:T2)  [unwired: 5 in, 2 out]
                n308 = To Long Integer(number=w314) -> (32bit integer=w313:i32)
                n309 = call-poly <vilib>:"Write Key.vi"("section"=w312, "value"=w313, "key"="Algorithm switch time", "refnum"=w317) -> ("refnum out"=w316:T2)  [unwired: 5 in, 2 out]
                n310 = call <vilib>:"Close Config Data.vi"("refnum"=w316) -> ("file path"=w324:path)  [unwired: 9 in, 1 out]
                n311 = Bundle("file path"=w324, TRUE) -> (w322:cluster{"file path":path, bool})  [unwired: 1 in]
                n312 = Enqueue Element(queue=w325, element=w322) -> ()  [unwired: 2 in, 3 out]
              }
            }
          }
          frame True {
            n313 = call "Display Message to User8"() -> ()  [unwired: 10 in, 2 out]
          }
        }
      }
      event "Restore configuration from file": Value Change {
        # "Ignore error"
        n314 = event-data() -> ()  [unwired: 1 in, 6 out]
        n315 = call "File Dialog2"("prompt"="Select configuration file to restore settings") -> ("selected path"=w382:path, "exists"=w381:bool, "cancelled"=w379:bool, "error out"=w377:errorcluster)  [unwired: 11 in]
        n316 = Unbundle By Name(w377) -> ()  [unwired: 1 out]
        n317 = Not(x=w379) -> (.not. x?=w378:bool)
        n318 = And(x=w381, y=w378) -> (x .and. y?=w380:bool)
        n319 = case shown="True" w380 {
          tunnel: w382 -> [_ w386]
          tunnel: w376 -> [_ w385]
          tunnel: w375 -> [_ w384]
          frame False {
            n320 = call "Display Message to User10"() -> ()  [unwired: 10 in, 2 out]
          }
          frame True {
            n321 = call "Display Message to User11"() -> ("Yes"=w387:bool)  [unwired: 10 in, 1 out]
            n322 = case shown="True" w387 {
              tunnel: w386 -> [_ w478]
              tunnel: w385 -> [_ w405]
              tunnel: w384 -> [_ w398]
              frame False {
              }
              frame True {
                w394 = "Controller" ("section")
                # "WTF is this"
                # "See the comment on the \"Save configuration file\" for some\ninformation about the format used. This one is even more\ntedious, since we have to make sure to provide default values\nso that LabVIEW doesn't mess up any controls that didn't\nhave values in the configuration file. This may not be terribly\nimportant now, but it'll be very nice if we ever add more\nstuff to the configuration file (since loading old configuration\nfiles won't break things)."
                n323 = property on="Step size (rev)" class="DigNum (strict)"() -> ("Value"=w474:dbl)  [unwired: 2 in, 2 out]
                n324 = call <vilib>:"Open Config Data.vi"("create file if necessary (T)"=FALSE, "configuration file path"=w478) -> ("refnum"=w476:T2)  [unwired: 7 in, 2 out]
                n325 = property on="Frequency to seek (GHz)" class="DigNum (strict)"() -> ("Value"=w470:dbl)  [unwired: 2 in, 2 out]
                n326 = call-poly <vilib>:"Read Key.vi"("section"=w394, "default value"=w474, "key"="Step size", "refnum"=w476) -> ("value"=w473:dbl, "found?"=w420:bool, "refnum out"=w472:T2)  [unwired: 4 in, 1 out]
                n327 = property on="Step size (rev)" class="DigNum (strict)"("Val(Sgnl)"=w473) -> ()  [unwired: 2 in, 2 out]
                n328 = call-poly <vilib>:"Read Key.vi"("section"=w394, "default value"=w470, "key"="Frequency to seek", "refnum"=w472) -> ("value"=w469:dbl, "found?"=w419:bool, "refnum out"=w468:T2)  [unwired: 4 in, 1 out]
                n329 = property on="Slope" class="DigNum (strict)"() -> ("Value"=w466:dbl)  [unwired: 2 in, 2 out]
                n330 = property on="Frequency to seek (GHz)" class="DigNum (strict)"("Value"=w469) -> ()  [unwired: 2 in, 2 out]
                n331 = call-poly <vilib>:"Read Key.vi"("section"=w394, "default value"=w466, "key"="Slope", "refnum"=w468) -> ("value"=w465:dbl, "found?"=w418:bool, "refnum out"=w464:T2)  [unwired: 4 in, 1 out]
                n332 = property on="Slope" class="DigNum (strict)"("Value"=w465) -> ()  [unwired: 2 in, 2 out]
                n333 = property on="Intercept" class="DigNum (strict)"() -> ("Value"=w462:dbl)  [unwired: 2 in, 2 out]
                n334 = property on="Automatic step size (rev)" class="DigNum (strict)"() -> ("Value"=w458:dbl)  [unwired: 2 in, 2 out]
                n335 = call-poly <vilib>:"Read Key.vi"("section"=w394, "default value"=w462, "key"="Intercept", "refnum"=w464) -> ("value"=w461:dbl, "found?"=w417:bool, "refnum out"=w460:T2)  [unwired: 4 in, 1 out]
                n336 = property on="Automatic velocity (rev/sec)" class="DigNum (strict)"() -> ("Value"=w454:dbl)  [unwired: 2 in, 2 out]
                n337 = property on="Intercept" class="DigNum (strict)"("Value"=w461) -> ()  [unwired: 2 in, 2 out]
                n338 = call-poly <vilib>:"Read Key.vi"("section"=w394, "default value"=w458, "key"="Automatic step size", "refnum"=w460) -> ("value"=w457:dbl, "found?"=w416:bool, "refnum out"=w456:T2)  [unwired: 4 in, 1 out]
                n339 = property on="Data input file" class="Path"() -> ("Text.Text"=w450:string)  [unwired: 2 in, 2 out]
                n340 = property on="Automatic step size (rev)" class="DigNum (strict)"("Value"=w457) -> ()  [unwired: 2 in, 2 out]
                n341 = property on="Seek positive polarization" class="Bool (strict)"() -> ("Value"=w434:bool)  [unwired: 2 in, 2 out]
                n342 = call-poly <vilib>:"Read Key.vi"("section"=w394, "default value"=w454, "key"="Automatic velocity", "refnum"=w456) -> ("value"=w453:dbl, "found?"=w415:bool, "refnum out"=w452:T2)  [unwired: 4 in, 1 out]
                n343 = property on="Automatic velocity (rev/sec)" class="DigNum (strict)"("Value"=w453) -> ()  [unwired: 2 in, 2 out]
                n344 = call-poly <vilib>:"Read Key.vi"("section"=w394, "default value"=w450, "key"="Data input file", "refnum"=w452) -> ("value"=w449:string, "found?"=w414:bool, "refnum out"=w448:T2)  [unwired: 4 in, 1 out]
                n345 = property on="Data input file" class="Path"("Text.Text"=w449) -> ()  [unwired: 2 in, 2 out]
                n346 = call-poly <vilib>:"Read Key.vi"("section"=w394, "default value"=w434, "key"="Seek positive", "refnum"=w448) -> ("value"=w433:bool, "found?"=w413:bool, "refnum out"=w447:T2)  [unwired: 4 in, 1 out]
                n347 = property on="Seek positive polarization" class="Bool (strict)"("Value"=w433) -> ()  [unwired: 2 in, 2 out]
                n348 = property on="Minimum" class="DigNum (strict)"() -> ("Value"=w431:dbl)  [unwired: 2 in, 2 out]
                n349 = call-poly <vilib>:"Read Key.vi"("section"=w394, "default value"=w431, "key"="Negative minimum frequency", "refnum"=w447) -> ("value"=w432:dbl, "found?"=w412:bool, "refnum out"=w446:T2)  [unwired: 4 in, 1 out]
                n350 = property on="Minimum" class="DigNum (strict)"("Value"=w432) -> ()  [unwired: 2 in, 2 out]
                n351 = property on="Maximum" class="DigNum (strict)"() -> ("Value"=w430:dbl)  [unwired: 2 in, 2 out]
                n352 = call-poly <vilib>:"Read Key.vi"("section"=w394, "default value"=w430, "key"="Negative maximum frequency", "refnum"=w446) -> ("value"=w429:dbl, "found?"=w411:bool, "refnum out"=w445:T2)  [unwired: 4 in, 1 out]
                n353 = property on="Maximum" class="DigNum (strict)"("Value"=w429) -> ()  [unwired: 2 in, 2 out]
                n354 = property on="Minimum" class="DigNum (strict)"() -> ("Value"=w427:dbl)  [unwired: 2 in, 2 out]
                n355 = call-poly <vilib>:"Read Key.vi"("section"=w394, "default value"=w427, "key"="Positive minimum frequency", "refnum"=w445) -> ("value"=w428:dbl, "found?"=w410:bool, "refnum out"=w444:T2)  [unwired: 4 in, 1 out]
                n356 = property on="Minimum" class="DigNum (strict)"("Value"=w428) -> ()  [unwired: 2 in, 2 out]
                n357 = property on="Maximum" class="DigNum (strict)"() -> ("Value"=w425:dbl)  [unwired: 2 in, 2 out]
                n358 = call-poly <vilib>:"Read Key.vi"("section"=w394, "default value"=w425, "key"="Positive maximum frequency", "refnum"=w444) -> ("value"=w426:dbl, "found?"=w409:bool, "refnum out"=w443:T2)  [unwired: 4 in, 1 out]
                n359 = property on="Maximum" class="DigNum (strict)"("Value"=w426) -> ()  [unwired: 2 in, 2 out]
                n360 = property on="Positive" class="DigNum (strict)"() -> ("Value"=w423:dbl)  [unwired: 2 in, 2 out]
                n361 = call-poly <vilib>:"Read Key.vi"("section"=w394, "default value"=w423, "key"="Positive home", "refnum"=w443) -> ("value"=w424:dbl, "found?"=w408:bool, "refnum out"=w442:T2)  [unwired: 4 in, 1 out]
                n362 = property on="Positive" class="DigNum (strict)"("Value"=w424) -> ()  [unwired: 2 in, 2 out]
                n363 = property on="Negative" class="DigNum (strict)"() -> ("Value"=w422:dbl)  [unwired: 2 in, 2 out]
                n364 = property on="Algorithm switch time (min)" class="DigNum (strict)"() -> ("Value"=w389:i64)  [unwired: 2 in, 2 out]
                n365 = call-poly <vilib>:"Read Key.vi"("section"=w394, "default value"=w422, "key"="Negative home", "refnum"=w442) -> ("value"=w421:dbl, "found?"=w407:bool, "refnum out"=w401:T2)  [unwired: 4 in, 1 out]
                n366 = property on="Negative" class="DigNum (strict)"("Value"=w421) -> ()  [unwired: 2 in, 2 out]
                n367 = call-poly <vilib>:"Read Key.vi"("section"=w394, "key"="Power data", "refnum"=w401) -> ("value"=w397:string, "found?"=w400:bool, "refnum out"=w396:T2)  [unwired: 5 in, 1 out]
                n368 = To Long Integer(number=w389) -> (32bit integer=w388:i32)
                n369 = in-place {
                  in-place-border: w397 -> [w480]
                  n370 = in-place-dvr #5(w398) -> (w481:refnum<class "Power control.lvclass">)  [unwired: 1 out]
                  n371 = call "From string.vi"("String"=w480, "Power control in"=w481) -> ("Power control out"=w479:refnum<class "Power control.lvclass">)  [unwired: 8 in, 1 out]
                  n372 = in-place-dvr #5(w479) -> ()  [unwired: 2 out]
                }
                n373 = call-poly <vilib>:"Read Key.vi"("section"=w394, "default value"=w388, "key"="Algorithm switch time", "refnum"=w396) -> ("value"=w390:i32, "found?"=w392:bool, "refnum out"=w395:T2)  [unwired: 4 in, 1 out]
                n374 = To Quad Integer(1:w390) -> (0:w391:i64)
                n375 = call <vilib>:"Close Config Data.vi"("refnum"=w395) -> ("file path"=w404:path)  [unwired: 9 in, 1 out]
                n376 = Compound Arithmetic op=AND(w420, w419, w418, w417, w416, w415, w414, w413, w412, w411, w410, w409, w408, w407, w400, w392) -> (w406:bool)
                n377 = property on="Algorithm switch time (min)" class="DigNum (strict)"("Value"=w391) -> ()  [unwired: 2 in, 2 out]
                n378 = case shown="False" w406 {
                  frame False {
                    n379 = call "Display Message to User16"() -> ()  [unwired: 10 in, 2 out]
                  }
                  frame True {
                  }
                }
                n380 = Bundle("file path"=w404, FALSE) -> (w403:cluster{"file path":path, bool})  [unwired: 1 in]
                n381 = Enqueue Element(queue=w405, element=w403) -> ()  [unwired: 2 in, 3 out]
              }
            }
          }
        }
      }
      event "Reset everything": Value Change {
        n382 = event-data() -> ()  [unwired: 1 in, 6 out]
        n383 = Two Button Dialog(message="Are you sure you want to completely reset all program data and stop communication? You will have to recalibrate frequencies, and the current automatic seek mode state will be forgotten. Additionally, this will not move the motor back to a known position, so if you restart the motor after doing this, all saved frequency calibrations will be invalidated.", 1:"Nah, nevermind" ("F button name (\"Cancel\")"), 2:"DO IT" ("T button name (\"OK\")")) -> (T button?=w482:bool)
        n384 = case shown="True" w482 {
          tunnel: w486 -> [_ w487]
          frame False {
          }
          frame True {
            n385 = flat-sequence {
              tunnel: w487 -> [w489]
              frame #0 {
                n386 = control-ref of="This VI"() -> (w488:refnum<vi>)
                n387 = invoke class="VI" method="Default Vals.Reinit All"(reference=w488) -> ()  [unwired: 2 in, 3 out]
              }
              frame #1 {
                n388 = call "Signal.vi"("Signaller in"=w489) -> ()  [unwired: 9 in, 2 out]
              }
            }
          }
        }
      }
      event "Stop communication": Value Change {
        # "Move motor back to a known position (position 0)"
        n389 = event-data() -> ()  [unwired: 1 in, 5 out]
        n390 = property on="Motor position (rev)" class="DigNum (strict)"() -> ("Value"=w493:dbl)  [unwired: 2 in, 2 out]
        n391 = Negate(x=w493) -> (-x=w492:dbl)
        n392 = call-dynamic "Move.vi"("Amount (rev)"=w492, "Motor in"=w491) -> ("error out"=w490:errorcluster)  [unwired: 8 in, 1 out]
        n393 = call "Signal.vi"("error in (no error)"=w490, "Signaller in"=w494) -> ()  [unwired: 8 in, 2 out]
      }
      event Timeout {
        n394 = event-data() -> ()  [unwired: 1 in, 2 out]
      }
    }
  }
  n395 = while {
    tunnel: w10 -> [w497]
    shift-right: [w503] -> _
    shift-left: w41 -> [w504]
    tunnel: w29 -> [w502]
    shift-right: [w495] -> _
    shift-left: w37 -> [w496]
    stop <- w508 stop-if-true
    n396 = call "Peek or default.vi"("Signaller in"=w497) -> ("Has signal?"=w508:bool)  [unwired: 8 in, 2 out]
    n397 = property on="Automatic mode on/off" class="Bool (strict)"() -> ("Value"=w501:bool)  [unwired: 2 in, 2 out]
    n398 = case shown="True" w501 {
      tunnel: "Data input file" -> [w510 w516]
      tunnel: [w510 w513] -> w499
      tunnel: [FALSE ("Filepath valid?") w514] -> w498
      frame False {
      }
      frame True {
        # "Prompt the user for a data filepath if none is selected"
        n399 = call "Select filepath if none.vi"("Error message"="Must select a data file to use automatic mode.", "Selector prompt"="Select a data file", "Filepath in"=w516) -> ("Filepath valid?"=w511:bool, "Filepath out"=w515:path)
        n400 = case shown="False" w511 {
          tunnel: w515 -> [_ w530]
          frame False {
            # "Turn off automatic mode so the user isn't\nprompted again and again"
            n401 = property on="Automatic mode on/off" class="Bool (strict)"("Val(Sgnl)"=FALSE ("Value (Signaling)")) -> ()  [unwired: 2 in, 2 out]
          }
          frame True {
            # "Update the filepath control to this\nnewly selected path"
            n402 = property on="Data input file" class="Path"("Value"=w530) -> ()  [unwired: 2 in, 2 out]
          }
        }
        n403 = case shown="True" w511 {
          tunnel: w515 -> [w520 w524]
          tunnel: [w520 w523] -> w513
          tunnel: [TRUE w521] -> w512
          frame False {
          }
          frame True {
            n404 = call <vilib>:"Check if File or Folder Exists.vi"("path"=w524) -> ("file or folder exists?"=w522:bool, "dup path"=w523:path)  [unwired: 8 in, 1 out]
            n405 = case shown="False" w522 {
              tunnel: [FALSE TRUE] -> w521
              frame False {
                n406 = call "Display Message to User17"() -> ("OK"=w526:bool)  [unwired: 10 in, 1 out]
                n407 = Not(x=w526) -> (.not. x?=w527:bool)
                n408 = property on="Automatic mode on/off" class="Bool (strict)"("Val(Sgnl)"=w527) -> ()  [unwired: 2 in, 2 out]
              }
              frame True {
              }
            }
          }
        }
        n409 = And(x=w512, y=w511) -> (x .and. y?=w514:bool)
      }
    }
    n410 = property on="Alarm" class="Bool (strict)"() -> ("Value"=w507:bool)  [unwired: 2 in, 2 out]
    n411 = Not(x=w507) -> (.not. x?=w506:bool)
    n412 = And(x=w498, y=w506) -> (x .and. y?=w505:bool)
    n413 = case shown="True" w505 {
      tunnel: w504 -> [w532 w546]
      tunnel: [w532 w545] -> w503
      tunnel: w502 -> [_ w544]
      tunnel: w499 -> [_ w542]
      tunnel: w497 -> [_ w541]
      tunnel: w496 -> [w531 w540]
      tunnel: [w531 w533] -> w495
      frame False {
      }
      frame True {
        w543 = u32 1000  # ms to wait between samples
        n414 = call "Get last row.vi"("Data input file"=w542) -> ("last row"=w539:string[])
        n415 = call "Input data row.vi"("Last row of data file"=w539, "Automatic Mode in"=w540) -> ("Automatic Mode out"=w538:refnum<class "Automatic Mode.lvclass">)  [unwired: 8 in, 1 out]
        n416 = call "Get number of samples taken.vi"("Automatic Mode in"=w538) -> ("Number of samples taken"=w537:i32, "Automatic Mode out"=w536:refnum<class "Automatic Mode.lvclass">)  [unwired: 8 in, 1 out]
        n417 = property on="Samples taken" class="DigNum (strict)"("Value"=w537) -> ()  [unwired: 2 in, 2 out]
        n418 = call "Has all samples.vi"("Automatic Mode in"=w536) -> ("Has all samples?"=w535:bool, "Automatic Mode out"=w534:refnum<class "Automatic Mode.lvclass">)  [unwired: 8 in, 1 out]
        n419 = Wait Until Next ms Multiple(millisecond multiple=w543) -> ()  [unwired: 1 out]
        n420 = case shown="True" w535 {
          tunnel: w546 -> [w548 w584]
          tunnel: [w548 w575] -> w545
          tunnel: w544 -> [_ w562]
          tunnel: w541 -> [_ w580]
          tunnel: w534 -> [w547 w579]
          tunnel: [w547 w555] -> w533
          frame False {
          }
          frame True {
            w581 = 5  # Seconds to wait
            w576 = 0  # Reset array pos to 0
            # "Check to see if the position we want to\nmove to is within bounds"
            # "Move in the appropriate direction (true means \"move up\") using the appropriate distance; the direction and distance are determined by the results of the previous conditional comparing the old and new rates (the \"step size\" is the distance)."
            # "Change directions if the rate at this position\nisn't at least as good as the last one"
            # "Give the motor some time;\nwe use the \"wait\" method\nof the stop notifier so that\nwe can still be listening for\nstop notifications while we wait.\nThis means that the user can\nstop the VI and not have to\nwait 5 seconds for this delay\nto finish (it'll stop within 100ms\nor so)."
            n421 = call "Get last data point.vi"("Automatic Mode in"=w579) -> ("Polarization"=w556:dbl, "Eventnum"=w578:i64, "Automatic Mode out"=w577:refnum<class "Automatic Mode.lvclass">)  [unwired: 7 in, 1 out]
            n422 = call "Decide next action.vi"("Polarization-based seek? (F)"="Polarization seek", "\"Good\" rate threshold"="\"Good\" rate threshold", "Seek positive polarization?"="Seek positive polarization", "Automatic Mode in"=w577) -> ("Calculated rate"=w550:dbl, "Decision"=w551:T3, "Automatic Mode out"=w555:refnum<class "Automatic Mode.lvclass">, "Should reseek?"=w549:bool)  [unwired: 3 in, 1 out]
            n423 = flat-sequence {
              tunnel: w556 -> [w599]
              tunnel: w550 -> [w600]
              tunnel: w578 -> [w601]
              frame #0 {
                # "Update the data points on the front panel"
                "Polarization" <- w599
                "Rate" <- w600
              }
              frame #1 {
                # "The eventnum must be updated last to maintain\ncompatibility with the grapher, which expects\nit to be the last value updated"
                "Eventnum" <- w601
              }
            }
            n424 = case shown="\"No motion\"" w551 {
              tunnel: w584 -> [w610 w616 w617]
              tunnel: [w609 w616 w617] -> w567
              tunnel: "Step size (rev)" -> [w606 w615 _]
              tunnel: [w605 w615 0.0 ("Step size (rev)")] -> w583
              frame "Switch direction" {
                w608 = 0.001  # Minimum step size
                # "Change directions and adjust step size"
                n425 = Greater?(x=w606, y=w608) -> (0:w607:bool)
                n426 = case shown="True" w607 {
                  tunnel: w606 -> [w611 w613]
                  tunnel: [w611 w612] -> w605
                  frame False {
                  }
                  frame True {
                    w614 = 0.9  # Step size diminuation factor
                    n427 = Multiply(x=w613, y=w614) -> (x*y=w612:dbl)
                  }
                }
                n428 = Not(x=w610) -> (.not. x?=w609:bool)
                n429 = property on="Step size (rev)" class="DigNum (strict)"("Value"=w605) -> ()  [unwired: 2 in, 2 out]
              }
              frame "Keep current direction" {
              }
              frame "No motion" {
              }
            }
            n430 = case shown="True" w549 {
              frame False {
              }
              frame True {
                n431 = property on="Reseek" class="Bool (strict)"("Val(Sgnl)"=TRUE ("Value (Signaling)")) -> ()  [unwired: 2 in, 2 out]
              }
            }
            n432 = property on="Home frequency" class="Clust (strict)"() -> ("Value"=w570:cluster{"Positive":dbl, "Negative":dbl})  [unwired: 2 in, 2 out]
            n433 = Unbundle By Name(w570) -> ("Positive"=w569:dbl, "Negative"=w568:dbl)
            n434 = case shown="False" "Seek positive polarization" {
              tunnel: ["Negative seek bounds" "Positive seek bounds"] -> w574
              tunnel: w569 -> [_ w597]
              tunnel: [w595 w597] -> w558
              tunnel: w568 -> [w595 _]
              frame False {
              }
              frame True {
              }
            }
            n435 = case shown="True" w567 {
              tunnel: w583 -> [w603 w604]
              tunnel: [w602 w604] -> w564
              frame False {
                n436 = Negate(x=w603) -> (-x=w602:dbl)
              }
              frame True {
              }
            }
            n437 = call-dynamic "Get position.vi"("Motor in"=w562) -> ("Position (rev)"=w565:dbl, "Motor out"=w561:refnum<class "Motor.lvclass">)  [unwired: 8 in, 1 out]
            n438 = property on="Fit parameters" class="Clust (strict)"() -> ("Value"=w557:cluster{"Slope":dbl, "Intercept":dbl})  [unwired: 2 in, 2 out]
            n439 = Add(x=w565, y=w564) -> (x+y=w563:dbl)
            n440 = Unbundle(w574) -> ("Minimum"=w573:dbl, "Maximum"=w572:dbl)
            n441 = call "Motor position to frequency.vi"("Fit parameters"=w557, "Motor position"=w563) -> ("Frequency"=w566:dbl)  [unwired: 9 in]
            n442 = In Range and Coerce(upper limit=w572, x=w566, lower limit=w573) -> (In Range?=w560:bool)  [unwired: 1 out]
            n443 = Not(x=w560) -> (.not. x?=w571:bool)
            n444 = case shown="False" w560 {
              tunnel: w561 -> [w588 w594]
              tunnel: w564 -> [_ w593]
              tunnel: [w589 w592] -> w559
              tunnel: w558 -> [w587 _]
              tunnel: w557 -> [w586 _]
              frame False {
                # "We should also reset the\nstep size, so we can try to\nfind a better position in the\nfuture"
                # "Go back to home position\nif we went out of bounds"
                n445 = call "Frequency to motor position.vi"("Fit parameters"=w586, "Frequency"=w587) -> ("Motor position"=w590:dbl)  [unwired: 9 in]
                n446 = property on="Automatic step size (rev)" class="DigNum (strict)"() -> ("Value"=w591:dbl)  [unwired: 2 in, 2 out]
                n447 = property on="Step size (rev)" class="DigNum (strict)"("Value"=w591) -> ()  [unwired: 2 in, 2 out]
                n448 = call-dynamic "Move to position.vi"("Position"=w590, "Motor in"=w588) -> ("error out"=w589:errorcluster)  [unwired: 8 in, 1 out]
              }
              frame True {
                n449 = call-dynamic "Move.vi"("Amount (rev)"=w593, "Motor in"=w594) -> ("error out"=w592:errorcluster)  [unwired: 8 in, 1 out]
              }
            }
            n450 = Exclusive Or(1:w571, 2:w567) -> (0:w575:bool)
            n451 = call "Wait on signal.vi"("error in (no error)"=w559, "Seconds to wait"=w581, "Signaller in"=w580) -> ()  [unwired: 7 in, 2 out]
            "Samples taken" <- w576
          }
        }
      }
    }
  }
  n452 = case shown="True" w33 {
    frame False {
    }
    frame True {
      n453 = call "Display Message to User2"() -> ("Thanks, I'll try that"=w619:bool)  [unwired: 10 in, 1 out]
      n454 = Stop(stop? (T)=w619) -> ()
    }
  }
  n455 = property on="Debug mode" class="Bool (strict)"("DisabledEnum"=w3) -> ()  [unwired: 2 in, 2 out]
  n456 = property on="Samples per step" class="DigNum (strict)"("DisabledEnum"=w3) -> ()  [unwired: 2 in, 2 out]
  n457 = property on="COM Port" class="VISAName"("DisabledEnum"=w3) -> ()  [unwired: 2 in, 2 out]
  n458 = property on="Reseek after # bad" class="DigNum (strict)"("DisabledEnum"=w3) -> ()  [unwired: 2 in, 2 out]
  n459 = call-dynamic "Destroy.vi"("Motor in"=w27) -> ()  [unwired: 10 in, 1 out]
  n460 = call "Destroy.vi"("Signaller in"=w42) -> ("error out"=w40:errorcluster)  [unwired: 10 in]
  n461 = flat-sequence {
    tunnel: w40 -> [_]
    frame #0 {
      # "Turn automatic mode off when the VI is stopped;\nthat way, it doesn't try to start in automatic\nmode immediately on the next startup"
      n462 = property on="Automatic mode on/off" class="Bool (strict)"("Val(Sgnl)"=FALSE ("Automatic mode on/off")) -> ()  [unwired: 2 in, 2 out]
    }
  }
